vi "Generate Debugging Disabled String.vi"(8 "error in (no error)":errorcluster, 11 "Coverage Analyzer Result View in":refnum<class "Coverage Analyzer Result View.lvclass">) -> (0 "error out":errorcluster, 2 "Disabled Debuggin":string, 3 "Coverage Analyzer Result View out":refnum<class "Coverage Analyzer Result View.lvclass">)   [LabVIEW 2020, in "Coverage Analyzer Result View.lvclass"]
uses:
  Coverage Analyzer Result View.lvclass
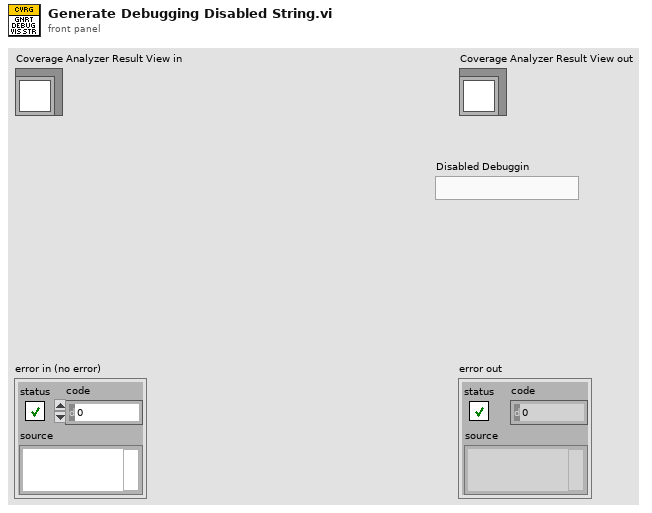
[diagram p1: front panel]
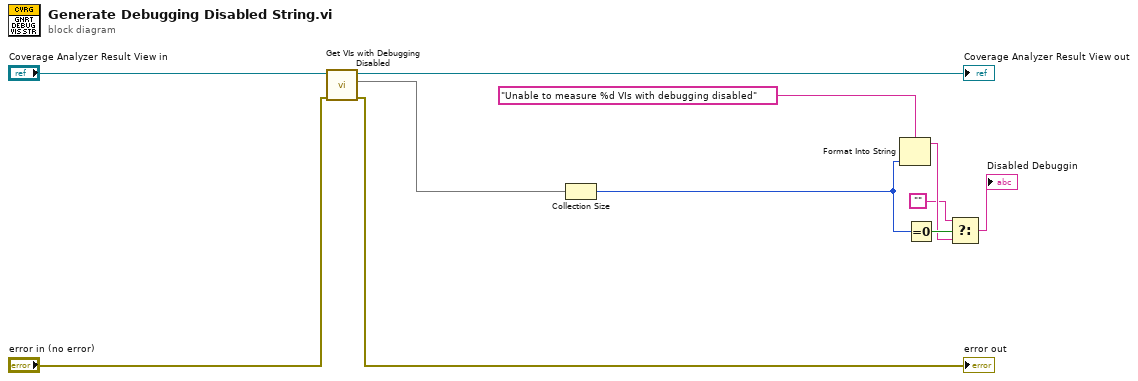
[diagram p0: block diagram]
diagram:
  n1 = call "Get VIs with Debugging Disabled.vi"("error in (no error)"="error in (no error)", "Coverage Analyzer Result View in"="Coverage Analyzer Result View in") -> ("error out"=→"error out":errorcluster, "VIs"=w6:set{path}, "Coverage Analyzer Result View out"=→"Coverage Analyzer Result View out":refnum<class "Coverage Analyzer Result View.lvclass">)  [unwired: 7 in]
  n2 = Collection Size(1:w6) -> (0:w4:i32)
  n3 = Format Into String(format string="Unable to measure %d VIs with debugging disabled", w4) -> (resulting string=w3:string)  [unwired: 2 in, 1 out]
  n4 = Equal To 0?(x=w4) -> (x = 0?=w5:bool)
  n5 = Select(t="", s=w5, f=w3) -> (s? t:f=→"Disabled Debuggin":string)
